vi "SVL Measure Propagation Delay (DAQmx).vi"(0 "output configuration":T5={"AO physical channel"="", "max value (3.5 V)"=3.5, "min value (-3.5 V)"=-3.5, "terminal configuration"=-1} {"terminal configuration" items=["Default"=-1, "RSE"=10083, "Differential"=10106, "Pseudodifferential"=12529]; "min value (-3.5 V)" format="%.2f"; "max value (3.5 V)" format="%.2f"}, 1 "input configuration":T4={"AI physical channel"="", "max value (3.5 V)"=3.5, "min value (--3.5 V)"=-3.5, "terminal configuration"=-1, "DSA channel settings"={"coupling"=10050, "enable IEPE excitation"=FALSE, "IEPE current [mA]"=4.0}} {"DSA channel settings"."IEPE current [mA]" format="%.1f"; "DSA channel settings"."coupling" items=["AC"=10045, "DC"=10050, "GND"=10066]; "terminal configuration" items=["Default"=-1, "RSE"=10083, "NRSE"=10078, "Differential"=10106, "Pseudodifferential"=12529]; "min value (--3.5 V)" format="%.2f"; "max value (3.5 V)" format="%.2f"}, 2 "maximum propagation delay [samples]":i32=150 min=2 step=1, 3 "number of averages":i32=10, 4 "sample frequency [Hz]":dbl=50000.0 min=1.0 format="%.2f", 5 "error in (no error)":errorcluster, 6 "test signal":u16(ring) items=["Smooth pulse"=0, "MLS"=10, "Chirp"=11], 8 "smooth pulse parameters":T2={"pulse width [samples]"=20, "amplitude [V peak]"=1.4} {"amplitude [V peak]" format="%.2p"; "pulse width [samples]" min=6 step=1}, 10 "broadband parameters":cluster{"amplitude [V peak]":dbl}={"amplitude [V peak]"=1.4} {"amplitude [V peak]" format="%.2p"}) -> (14 "Generated and Acquired Waveforms":waveform(dbl)[](graph) caption="generated and acquired waveforms", 16 "average propagation delay [samples]":dbl format="%.2f", 17 "Propagation Delay":dbl[](graph) caption="propagation delay [samples]", 19 "error out":errorcluster)   [LabVIEW 2017, in "SoundVib_Calibration.lvlib"]
doc: "Measures the propagation delay of the measurement hardware and the device under test (DUT). You can measure the propagation delay of the device under test by subtracting the propagation delay of the measurement system without the DUT from the measured propagation delay of the entire system, including the DUT. The propagation delay is returned in number of samples. This VI uses the NI-DAQmx driver."
uses:
  <vilib>/addons/Sound and Vibration/svt_Calibration/SoundVib_Calibration.lvlib
  <vilib>/addons/_NISVFA/_Shared subVIs/Controls/svc_DSA Channel Settings.ctl
  <vilib>/addons/_NISVFA/_Shared subVIs/Controls/svc_Analog Level Trigger Configuration.ctl
  <vilib>/DAQmx/read.llb/DAQmx Read (Analog Wfm 1Chan NSamp).vi
  <vilib>/DAQmx/write.llb/DAQmx Write (Analog 1D DBL 1Chan NSamp).vi
  <vilib>/DAQmx/miscellaneous.llb/DAQmx Fill In Error Info.vi
  <vilib>/DAQmx/configure/timing.llb/DAQmx Timing (Sample Clock).vi
  <vilib>/DAQmx/create/channels.llb/DAQmx Create Channel (AI-Voltage-Basic).vi
  <vilib>/DAQmx/create/channels.llb/DAQmx Create Channel (AO-Voltage-Basic).vi
  <vilib>/Analysis/NI_AALBase.lvlib
  <vilib>/addons/_NISVFA/_Generation/SoundVib_Generation.lvlib
  <resource>/objmgr/daqmx.rc
panel:
  in  "Tab Control":T1(tab)=enum."Configuration"
  out "String":string="GETTING STARTED\n\nQuantifying the signal propagation delay is important in many applications involving stimulus and response testing. The propagation delay is the interval between when a sample is generated on the output of your measurement device and when the corresponding sample is acquired on the input side. Propagation delay can be expressed either in terms of samples or time (seconds). This VI expresses the delay in samples.\n\nSeveral of the Audio Measurement and Swept Sine example programs in the LabVIEW Sound and Vibration Toolset request the propagation delay as an input. If you do not know the propagation delay, the SVL Measure Propagation Delay VI provides a quick method to measure it.\n\nThe two main sources of propagation delay are signal propagation from the measurement device to and from the device under test (DUT) and the measurement device itself. In purely electrical systems, propagation delay caused by signal propagation from the measurement device to and from the DUT is often negligible unless you are testing at very high frequencies.  However, the delay is often significant in mechanical or acoustical tests. For example, if the DUT is a speaker, it is important to consider the time for sound to travel from the speaker to the microphone. An example of the measurement device being the source of the propagation delay is the brick wall anti-aliasing and anti-imaging filters on the NI PXI-4461 DSA devices which generate a total delay on the order of 100 samples. The delay on the 4461 is dependent on the sample rate, so you should measure the propagation delay at the same sample rate used in your measurement application.\n\nThe SVL Measure Propagation Delay VI measures the total delay from both sources, the DUT as well as the measurement device. If you would like to examine only the device propagation delay, you should short your input and output channels as shown in the upper wiring diagram. To measure the delay in the measurement device as well as time to and from the DUT, you should connect the DUT as shown in the lower wiring diagram. The lower diagram does not include any transducers that may be needed.\n\nThis VI generates an analog output signal (smooth pulse or MLS) and measures the delay between the generated signal and the acquired signal. The delay is returned in sample intervals under the \"Measurement Results\" tab."
  in  "stop":bool
  out "measurement progress":i32(slide) max=10 scale=0.0..10.0
  in  "update graphs":bool
  # "Measure propagation delay of DAQ/DSA device"
  # "Measuring system propagation delay  (DAQ/DSA device, transducers, and DUT)"
  # "DAQ Configuration"
  # "Measurement Configuration"
  # "total AO --> AI"
  # "Test Signal Configuration"
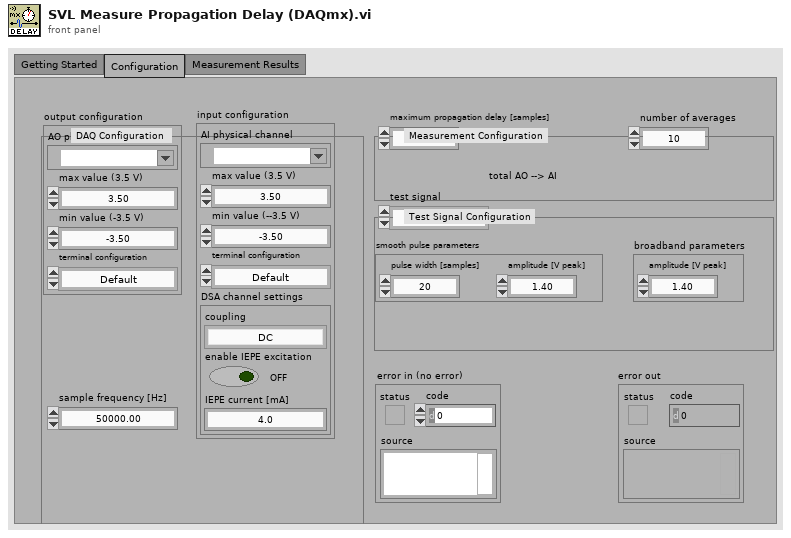
[diagram p1: front panel]
types:
  T1 = enum32{"Getting Started", "Configuration", "Measurement Results"}
  T2 = cluster{"pulse width [samples]":i32, "amplitude [V peak]":dbl}
  T3 = typedef "svc_DSA Channel Settings.ctl" = cluster{"coupling":i32, "enable IEPE excitation":bool, "IEPE current [mA]":dbl}
  T4 = cluster{"AI physical channel":tag, "max value (3.5 V)":dbl, "min value (--3.5 V)":dbl, "terminal configuration":i32, "DSA channel settings":T3}
  T5 = cluster{"AO physical channel":tag, "max value (3.5 V)":dbl, "min value (-3.5 V)":dbl, "terminal configuration":i32}
  T6 = typedef "svc_Analog Level Trigger Configuration.ctl" = cluster{"level":dbl, "slope":u16, "hysteresis":dbl}
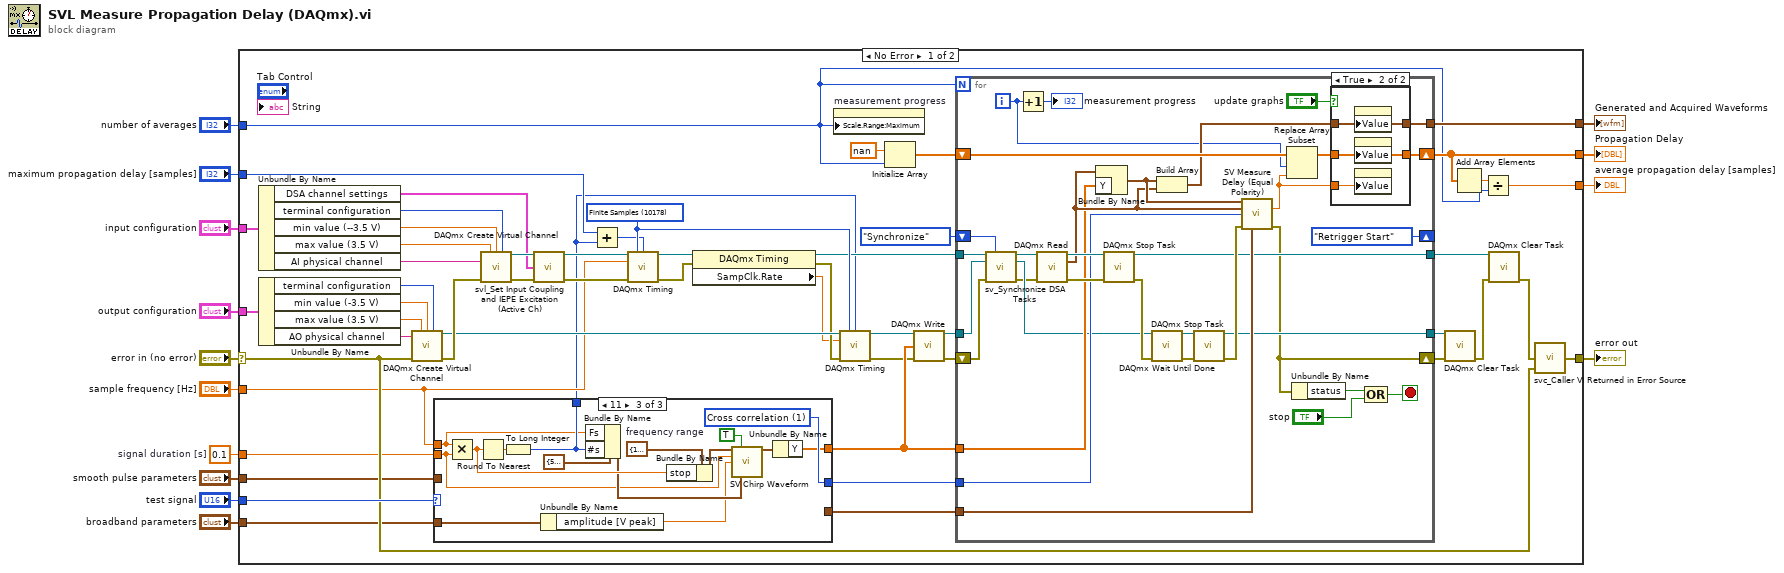
[diagram p0: block diagram]
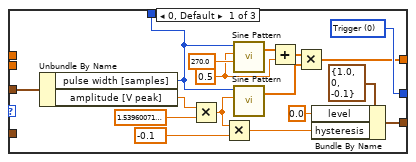
[diagram p3: hidden frame]
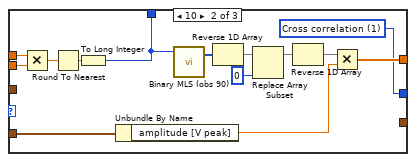
[diagram p4: hidden frame]
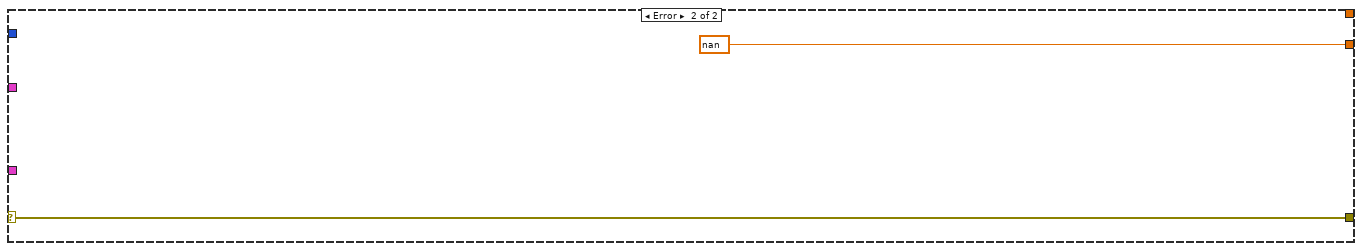
[diagram p5: hidden frame]
diagram:
  w3 = 0.1  # signal duration [s]
  n1 = case shown="No Error" "error in (no error)" {
    selector: "error in (no error)" -> [w47 w154]
    tunnel: [w46 w154] -> w4
    tunnel: "maximum propagation delay [samples]" -> [w32 _]
    tunnel: "number of averages" -> [w17 _]
    tunnel: "output configuration" -> [w62 _]
    tunnel: "input configuration" -> [w61 _]
    tunnel: "sample frequency [Hz]" -> [w30 _]
    tunnel: "test signal" -> [w51 _]
    tunnel: [w63 _] -> w7
    tunnel: [w54 _] -> w6
    tunnel: [w53 nan] -> w5
    tunnel: w3 -> [w20 _]
    tunnel: "smooth pulse parameters" -> [w16 _]
    tunnel: "broadband parameters" -> [w15 _]
    frame No Error {
      w33 = 10178 items=["Finite Samples"=10178, "Continuous Samples"=10123, "Hardware Timed Single Point"=12522] ("sample mode")
      n2 = Unbundle By Name(w61) -> ("DSA channel settings"=w42:T3, "terminal configuration"=w58:i32, "min value (--3.5 V)"=w57:dbl, "max value (3.5 V)"=w66:dbl, "AI physical channel"=w45:tag)
      n3 = Unbundle By Name(w62) -> ("terminal configuration"=w52:i32, "min value (-3.5 V)"=w67:dbl, "max value (3.5 V)"=w60:dbl, "AO physical channel"=w59:tag)
      n4 = call-poly <vilib>:"DAQmx Create Virtual Channel.vi"("maximum value"=w60, "minimum value"=w67, "output terminal configuration"=w52, "physical channels"=w59, "error in"=w47) -> ("task out"=w38:refnum<k21>, "error out"=w39:errorcluster)  [unwired: 9 in]
      n5 = case shown="11" w51 {
        tunnel: [w110 w137 w148] -> w40
        tunnel: [w108 w127 w144] -> w19
        tunnel: [w111 w136 w151] -> w49
        tunnel: [w114 _ _] -> w48
        tunnel: w30 -> [_ w130 w143]
        tunnel: w20 -> [_ w125 w141]
        tunnel: w16 -> [w107 _ _]
        tunnel: w15 -> [_ w124 w140]
        frame 0, Default {
          w111 = u16 0 items=["Trigger", "Cross correlation", "Phase lag"] ("method")
          w116 = 0.5 ("phase(degrees)")
          n6 = Unbundle By Name(w107) -> ("pulse width [samples]"=w108:i32, "amplitude [V peak]"=w115:dbl)
          n7 = Multiply(x=w115, y=1.539600717839002 ("1/x")) -> (x*y=w118:dbl)
          n8 = Multiply(x=w118, y=-0.1) -> (x*y=w113:dbl)
          n9 = call <vilib>:"Sine Pattern.vi"("phase(degrees)"=270.0, "amplitude"=w116, "samples"=w108) -> ("Sinusoidal Pattern"=w120:dbl[])  [unwired: 1 in, 1 out]
          n10 = call <vilib>:"Sine Pattern.vi"("amplitude"=w118, "samples"=w108) -> ("Sinusoidal Pattern"=w122:dbl[])  [unwired: 2 in, 1 out]
          n11 = Add(x=w120, y=w116) -> (x+y=w119:dbl[])
          n12 = Multiply(x=w119, y=w122) -> (x*y=w110:dbl[])
          n13 = Bundle By Name(cluster=T6 {"level"=1.0, "slope"=0, "hysteresis"=-0.1} ("trigger parameters"), "level"=0.0 ("Element Data"), "hysteresis"=w113) -> (w114:T6)
        }
        frame 10 {
          w136 = u16 1 items=["Trigger", "Cross correlation", "Phase lag"] ("method")
          n14 = Multiply(x=w130, y=w125) -> (x*y=w129:dbl)
          n15 = Round To Nearest(number=w129) -> (nearest integer value=w128:dbl)
          n16 = To Long Integer(number=w128) -> (32bit integer=w127:i32)
          n17 = Unbundle By Name(w124) -> ("amplitude [V peak]"=w126:dbl)
          n18 = call <vilib>:"Binary MLS (obs 90).vi"("samples"=w127) -> ("mls sequence"=w135:u8[])  [unwired: 2 in, 1 out]
          n19 = Reverse 1D Array(array=w135) -> (reversed array=w134:u8[])
          n20 = Replace Array Subset(array=w134, new element=u8 0 ("new element/subarray")) -> (w132:u8[])  [unwired: 1 in]
          n21 = Reverse 1D Array(array=w132) -> (reversed array=w131:u8[])
          n22 = Multiply(x=w131, y=w126) -> (x*y=w137:dbl[])
        }
        frame 11 {
          w151 = u16 1 items=["Trigger", "Cross correlation", "Phase lag"] ("method")
          w150 = cluster{"start":dbl, "stop":dbl} {"start"=1000.0, "stop"=20000.0}  # frequency range
          n23 = Multiply(x=w143, y=w141) -> (x*y=w145:dbl)
          n24 = Round To Nearest(number=w145) -> (nearest integer value=w149:dbl)
          n25 = To Long Integer(number=w149) -> (32bit integer=w144:i32)
          n26 = Unbundle By Name(w140) -> ("amplitude [V peak]"=w139:dbl)
          n27 = Bundle By Name(cluster=cluster{"Fs":dbl, "#s":u32} {"Fs"=51200.0, "#s"=1024} ("sampling info"), "Fs"=w143, "#s"=w144) -> (w142:cluster{"Fs":dbl, "#s":u32})
          n28 = Bundle By Name(cluster=w150, "stop"=w145) -> (w147:cluster{"start":dbl, "stop":dbl})
          n29 = call <vilib>:"SV Chirp Waveform.vi"("frequency range"=w147, "reset signal (F)"=TRUE, "chirp duration [s]"=w141, "amplitude"=w139, "sampling info"=w142) -> ("chirp signal"=w152:waveform(dbl))  [unwired: 8 in, 2 out]
          n30 = Unbundle By Name(w152) -> ("Y"=w148:dbl[])
        }
      }
      n31 = call-poly <vilib>:"DAQmx Create Virtual Channel.vi"("maximum value"=w66, "minimum value"=w57, "input terminal configuration"=w58, "physical channels"=w45, "error in"=w39) -> ("task out"=w44:refnum<k21>, "error out"=w43:errorcluster)  [unwired: 9 in]
      n32 = call <vilib>:"svl_Set Input Coupling and IEPE Excitation (Active Ch).vi"("AI task name"=w44, "DSA channel settings"=w42, "error in (no error)"=w43) -> ("dup AI task name"=w35:refnum<k21>, "error out"=w34:errorcluster)  [unwired: 11 in]
      n33 = Add(x=w32, y=w19) -> (x+y=w31:i32)
      n34 = call-poly <vilib>:"DAQmx Timing.vi"("task/channels in"=w35, "sample mode"=w33, "samples per channel"=w31, "rate"=w30, "error in"=w34) -> ("task out"=w29:refnum<k21>, "error out"=w28:errorcluster)  [unwired: 9 in]
      n35 = property class="DAQmx Timing"(reference=w29, error in=w28) -> (reference out=w27:refnum<k21>, error out=w25:errorcluster, "SampClk.Rate"=w21:dbl)
      n36 = property on="measurement progress" class="Slide (strict)"("Scale.Range:Maximum"=w17) -> ()  [unwired: 2 in, 2 out]
      n37 = call-poly <vilib>:"DAQmx Timing.vi"("task/channels in"=w38, "sample mode"=w33, "samples per channel"=w19, "rate"=w21, "error in"=w25) -> ("task out"=w37:refnum<k21>, "error out"=w36:errorcluster)  [unwired: 9 in]
      n38 = Initialize Array(nan ("element"), w17) -> (w64:dbl[])
      n39 = call-poly <vilib>:"DAQmx Write.vi"("task/channels in"=w37, "data"=w40, "error in"=w36) -> ("task out"=w41:refnum<k21>, "error out"=w26:errorcluster)  [unwired: 10 in, 1 out]
      n40 = for {
        N: w17 -> [_]
        tunnel: [w100] -> w63
        shift-right: [w99] -> w54
        shift-left: w64 -> [w101]
        tunnel: w41 -> [w77]
        tunnel: w27 -> [w74]
        tunnel: [w89] -> w56
        tunnel: [w83] -> w55
        tunnel: w40 -> [w78]
        tunnel: w49 -> [w84]
        tunnel: w48 -> [w90]
        shift-right: [w79] -> w24
        shift-left: w26 -> [w75]
        shift-right: [enum16{"Synchronize", "Retrigger Start"}."Retrigger Start" ("action")] -> _
        shift-left: enum16{"Synchronize", "Retrigger Start"}."Synchronize" ("action") -> [w70]
        i -> [w69]
        stop <- w80 stop-if-true
        n41 = call <vilib>:"sv_Synchronize DSA Tasks.vi"("master task in"=w74, "action"=w70, "slave task in"=w77, "error in (no error)"=w75) -> ("master task out"=w73:refnum<k21>, "slave task out"=w76:refnum<k21>, "error out"=w72:errorcluster)  [unwired: 9 in]
        n42 = Increment(x=w69) -> (x+1=→"measurement progress":i32)
        n43 = call-poly <vilib>:"DAQmx Read.vi"("task/channels in"=w73, "error in"=w72) -> ("task out"=w96:refnum<k21>, "data"=w81:waveform(dbl), "error out"=w95:errorcluster)  [unwired: 11 in]
        n44 = Bundle By Name(cluster=w81, "Y"=w78) -> (w82:waveform(dbl))
        n45 = call <vilib>:"DAQmx Stop Task.vi"("task/channels in"=w96, "error in"=w95) -> ("task out"=w83:refnum<k21>, "error out"=w85:errorcluster)  [unwired: 12 in]
        n46 = call <vilib>:"DAQmx Wait Until Done.vi"("task/channels in"=w76, "error in"=w85) -> ("task out"=w93:refnum<k21>, "error out"=w92:errorcluster)  [unwired: 12 in]
        n47 = Build Array(w82, w81) -> (w98:waveform(dbl)[])
        n48 = call <vilib>:"DAQmx Stop Task.vi"("task/channels in"=w93, "error in"=w92) -> ("task out"=w89:refnum<k21>, "error out"=w94:errorcluster)  [unwired: 12 in]
        n49 = call <vilib>:"SV Measure Delay (Equal Polarity).vi"("reference signal"=w82, "delayed signal"=w81, "method"=w84, "error in"=w94, "trigger parameters"=w90) -> ("delay [samples]"=w71:dbl, "error out"=w79:errorcluster)  [unwired: 8 in, 1 out]
        n50 = Replace Array Subset(array=w101, new element=w71, index=w69) -> (w97:dbl[])
        n51 = Unbundle By Name(w79) -> ("status"=w88:bool)
        n52 = case shown="True" "update graphs" {
          tunnel: w98 -> [w103 w106]
          tunnel: [w103 w106] -> w100
          tunnel: w97 -> [w102 w105]
          tunnel: [w102 w105] -> w99
          tunnel: w71 -> [_ w104]
          frame False {
          }
          frame True {
            n53 = property on="Generated and Acquired Waveforms" class="WFGraph (strict)"("Value"=w106) -> ()  [unwired: 2 in, 2 out]
            n54 = property on="Propagation Delay" class="WFGraph (strict)"("Value"=w105) -> ()  [unwired: 2 in, 2 out]
            n55 = property on="average propagation delay [samples]" class="DigNum (strict)"("Value"=w104) -> ()  [unwired: 2 in, 2 out]
          }
        }
        n56 = Compound Arithmetic op=OR(w88, "stop") -> (w80:bool)
      }
      n57 = call <vilib>:"DAQmx Clear Task.vi"("task in"=w56, "error in"=w24) -> ("error out"=w23:errorcluster)  [unwired: 13 in]
      n58 = Add Array Elements(numeric array=w54) -> (sum=w50:dbl)
      n59 = Divide(x=w50, y=w17) -> (x/y=w53:dbl)
      n60 = call <vilib>:"DAQmx Clear Task.vi"("task in"=w55, "error in"=w23) -> ("error out"=w22:errorcluster)  [unwired: 13 in]
      n61 = call <vilib>:"svc_Caller VI Returned in Error Source.vi"("warning input to caller"=w47, "error in (no error)"=w22) -> ("error out"=w46:errorcluster)  [unwired: 3 in]
    }
    frame Error {
    }
  }
  "error out" <- w4
  "average propagation delay [samples]" <- w5
  "Propagation Delay" <- w6
  "Generated and Acquired Waveforms" <- w7
